vi "Wait On Listener.vi"(8 "error in (no error)":errorcluster, 9 "timeout ms (5000)":i32=5000, 11 "dotNET Listener in":refnum<class "dotNET Listener.lvclass">) -> (0 "error out":errorcluster, 2 "Socket out":refnum<class "Socket.lvclass">, 3 "dotNET Listener out":refnum<class "dotNET Listener.lvclass">)   [LabVIEW 2013, in "dotNET SSL Socket.lvlib" / "dotNET Listener.lvclass"]
uses:
  dotNET Listener.lvclass
  <vilib>/MediaMongrels Ltd/WebSockets/Sockets/Socket/Socket.lvclass
  dotNET Listener.lvclass/dotNET Listener.ctl
  dotNET TCP Socket/dotNET TCP Socket.lvclass
panel:
  out "Pending":bool
  out "WaitOne":bool
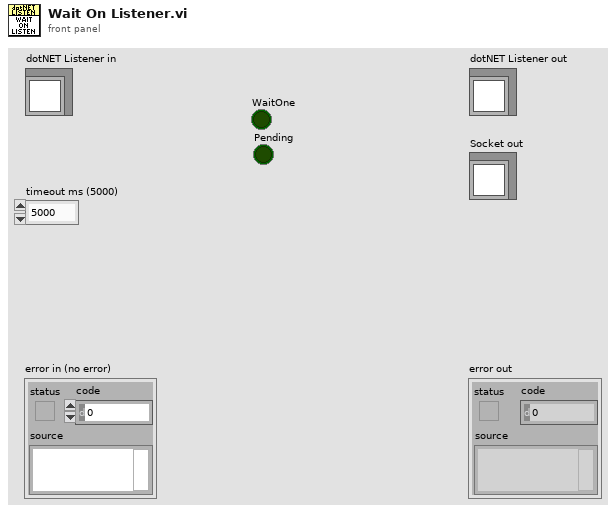
[diagram p1: front panel]
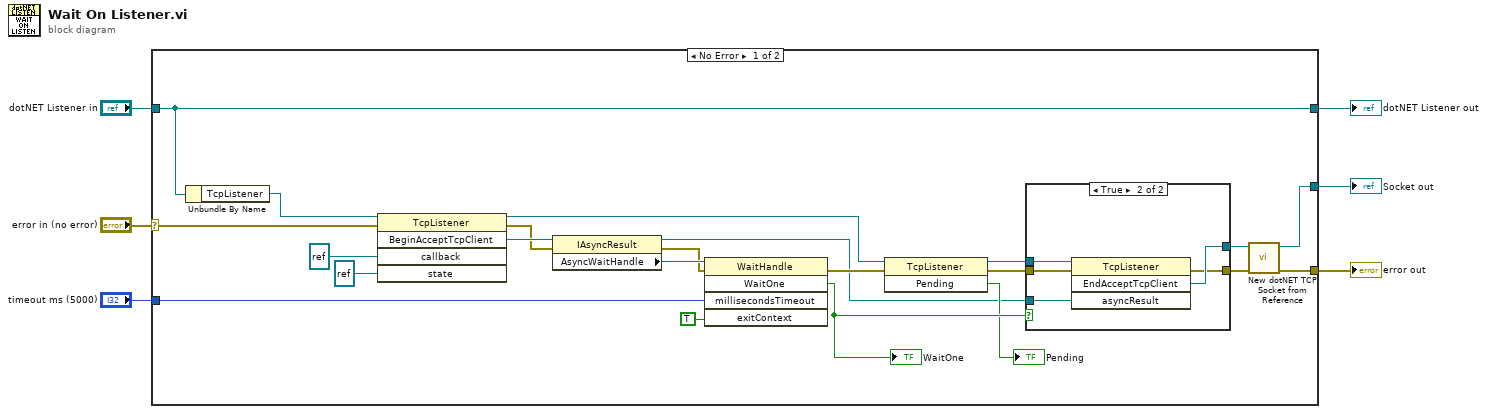
[diagram p0: block diagram]
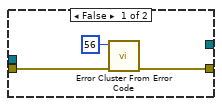
[diagram p2: hidden frame]
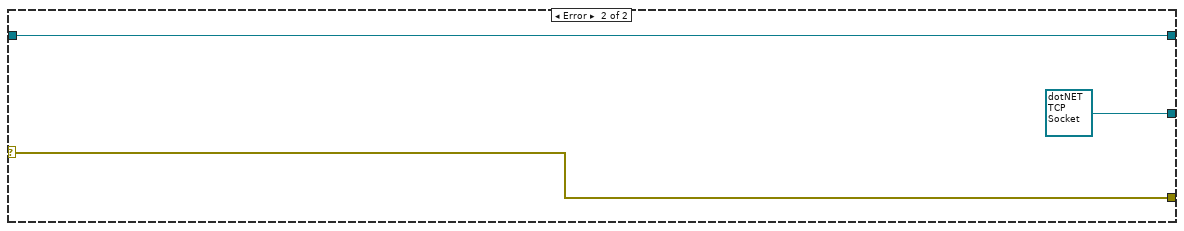
[diagram p3: hidden frame]
diagram:
  n1 = case shown="No Error" "error in (no error)" {
    selector: "error in (no error)" -> [w26 w39]
    tunnel: [w9 w39] -> w5
    tunnel: [w28 w38] -> w3
    tunnel: "dotNET Listener in" -> [w28 w38]
    tunnel: "timeout ms (5000)" -> [w25 _]
    tunnel: [w7 refnum<class "dotNET TCP Socket.lvclass"> refnum ("dotNET TCP Socket out")] -> w1
    frame No Error {
      n2 = Unbundle By Name(w28) -> ("TcpListener"=w27:refnum<k24>)
      n3 = invoke class="TcpListener" method="BeginAcceptTcpClient"(reference=w27, error in=w26, "callback"=refnum<k24> refnum, "state"=refnum<k24> refnum) -> (reference out=w19:refnum<k24>, error out=w17:errorcluster, "BeginAcceptTcpClient"=w24:refnum<k24>)  [unwired: 1 in, 2 out]
      n4 = property class="IAsyncResult"(reference=w24, error in=w17) -> (reference out=w12:refnum<k24>, error out=w14:errorcluster, "AsyncWaitHandle"=w23:refnum<k24>)
      n5 = invoke class="WaitHandle" method="WaitOne"(reference=w23, error in=w14, "millisecondsTimeout"=w25, "exitContext"=TRUE) -> (error out=w18:errorcluster, "WaitOne"=w16:bool)  [unwired: 1 in, 3 out]
      "WaitOne" <- w16
      n6 = invoke class="TcpListener" method="Pending"(reference=w19, error in=w18) -> (reference out=w11:refnum<k24>, error out=w13:errorcluster, "Pending"=→"Pending":bool)  [unwired: 1 in]
      n7 = case shown="True" w16 {
        tunnel: [_ w35] -> w8
        tunnel: [w31 w34] -> w10
        tunnel: w13 -> [w30 w36]
        tunnel: w12 -> [_ w33]
        tunnel: w11 -> [_ w32]
        frame False {
          n8 = call <vilib>:"Error Cluster From Error Code.vi"("error in (no error)"=w30, "error code (0)"=56) -> ("error out"=w31:errorcluster)  [unwired: 7 in]
        }
        frame True {
          n9 = invoke class="TcpListener" method="EndAcceptTcpClient"(reference=w32, error in=w36, "asyncResult"=w33) -> (error out=w34:errorcluster, "EndAcceptTcpClient"=w35:refnum<k24>)  [unwired: 1 in, 2 out]
        }
      }
      n10 = call "New dotNET TCP Socket from Reference.vi"("error in (no error)"=w10, "TcpClient"=w8) -> ("error out"=w9:errorcluster, "dotNET TCP Socket out"=w7:refnum<class "dotNET TCP Socket.lvclass">)  [unwired: 8 in]
    }
    frame Error {
    }
  }
  "error out" <- w5
  "dotNET Listener out" <- w3
  "Socket out" <- w1
